vi "RT.vi"() -> ()   [LabVIEW 2014]
uses:
  <vilib>/NI/LVFPGA Adv Session Resources/OpenByNameSubVI.vi
  <vilib>/FPGAPlugInAG/Dynamic/niLvFpga_Run_Dynamic.vi
  <vilib>/rvi/interface/common/dynamic/niFpgaEscapeDelimiterAndNull.vi
  <vilib>/Utility/error.llb/Error Cluster From Error Code.vi
  <vilib>/rvi/errors/niLvFpgaAdjustHostInterfaceError.vi
  <vilib>/FPGAPlugInAG/Dynamic/niLvFpga_Close_Dynamic.vi
  <vilib>/rvi/interface/nirviMethod/nirviMethod.xnode
  <vilib>/NI/LVFPGA Adv Session Resources/OpenByName.xnode
  <vilib>/rvi/interface/nirviReadWriteControl/nirviReadWriteControl.xnode
  <vilib>/rvi/interface/nirviCloseFPGA/nirviCloseFPGA.xnode
  <vilib>/FPGAPlugInAG/Dynamic/niLvFpga_WriteFifo_Dynamic.vi
  <vilib>/rvi/errors/niLvFpgaMergeErrorWithErrorCode.vi
  <vilib>/NI/LVFPGA Adv Session Resources/LVFPGAAdvSessionResources.lvlib
  NiFpgaLv.dll
  <vilib>/rvi/interface/Simulation/niFpgaSimulationCallBeginRW.vi
panel:
  out "Value":u32 format="%x"
  in  "Bitfile path":path=path "c:/ni-rt/LabVIEW Data/DETSPIExample_FPGATarget_SPIperipheral_T23U1l-two8.lvbitx"
  out "Empty Elements Remaining":u32=16383
  out "error out":errorcluster={"status"=FALSE, "code"=61003, "source"="niLvFpga_Run_Dynamic.vi"}
  in  "SPI command":u32=589824 format="%x"
  in  "Boolean":bool
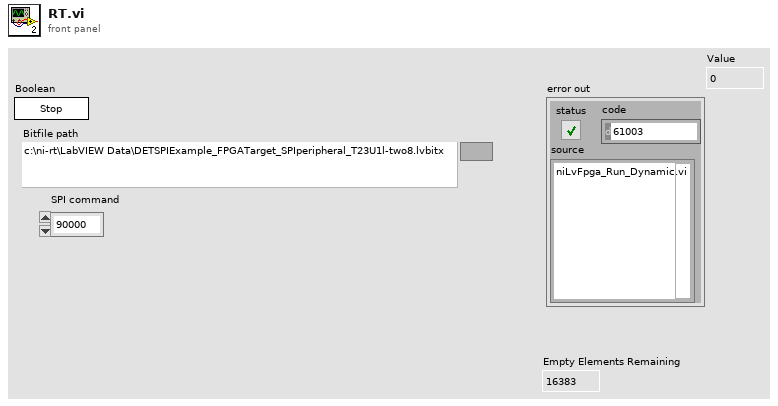
[diagram p1: front panel]
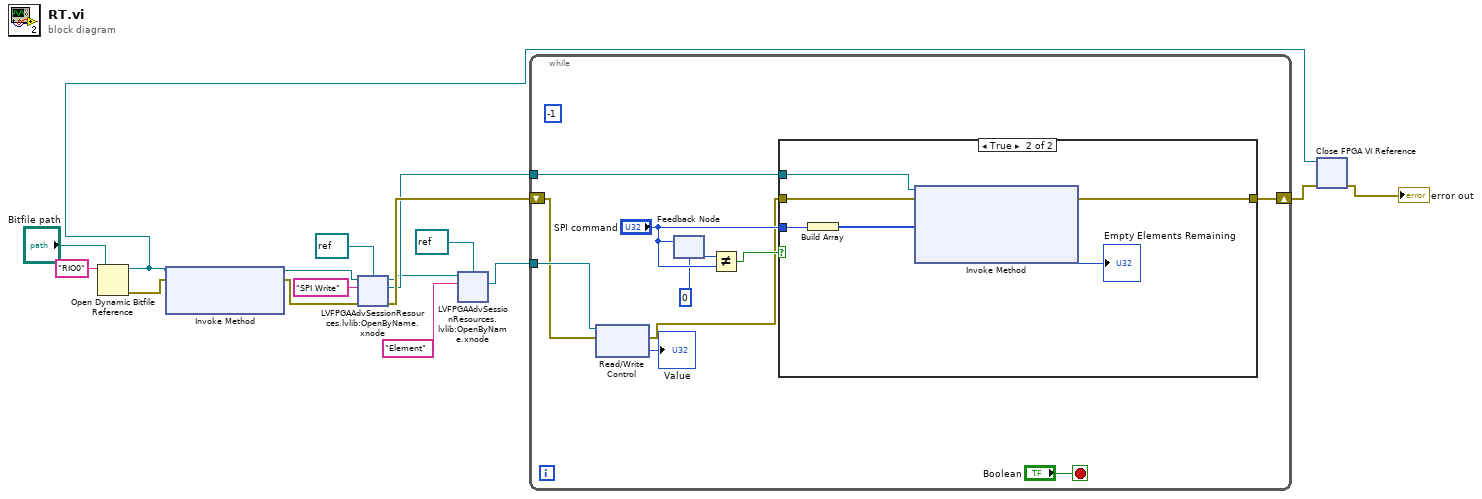
[diagram p0: block diagram]
diagram:
  n1 = Open Dynamic Bitfile Reference(0:"RIO0" ("Device address"), 1:"Bitfile path") -> (5:w11:refnum<k20>, 8:w14:errorcluster)  [unwired: 3 in]
  n2 = xnode "Invoke Method"("FPGA VI Reference In"=w11, "error in"=w14) -> ("FPGA VI Reference Out"=w5:refnum<k20>, "error out"=w8:errorcluster)  [unwired: 1 in]
  n3 = xnode "LVFPGAAdvSessionResources.lvlib:OpenByName.xnode"("FPGA VI Reference in"=w5, "Resource name in"="SPI Write", "Single resource reference type in"=refnum<k20> refnum, "Error in"=w8) -> ("Single resource reference out"=w6:refnum<k20>, "Error out"=w7:errorcluster, "FPGA VI Reference out"=w2:refnum<k20>)
  n4 = xnode "LVFPGAAdvSessionResources.lvlib:OpenByName.xnode"("FPGA VI Reference in"=w2, "Resource name in"="Element", "Single resource reference type in"=refnum<k20> refnum) -> ("Single resource reference out"=w1:refnum<k20>)  [unwired: 1 in, 2 out]
  n5 = while {
    tunnel: w6 -> [w21]
    shift-right: [w26] -> w13
    shift-left: w7 -> [w18]
    tunnel: w1 -> [w20]
    stop <- "Boolean" stop-if-true
    (unwired) -1
    n6 = xnode "Read/Write Control"("FPGA VI Reference In"=w20, "error in"=w18) -> ("error out"=w17:errorcluster, "Value"=→"Value":u32)  [unwired: 1 out]
    n7 = feedback-in #1("SPI command") -> ()
    n8 = feedback #1(u32 0 ("SPI command")) -> (w24:u32)
    n9 = Not Equal?(x=w24, y="SPI command") -> (x != y?=w22:bool)
    n10 = case shown="True" w22 {
      tunnel: w17 -> [w28 w32]
      tunnel: [w28 w31] -> w26
      tunnel: "SPI command" -> [_ w34]
      tunnel: w21 -> [_ w29]
      frame False {
      }
      frame True {
        n11 = Build Array(w34) -> (w33:u32[])
        n12 = xnode "Invoke Method"("FPGA VI Reference In"=w29, "error in"=w32, "Data"=w33) -> ("error out"=w31:errorcluster, "Empty Elements Remaining"=→"Empty Elements Remaining":u32)  [unwired: 1 in, 1 out]
      }
    }
  }
  n13 = xnode "Close FPGA VI Reference"("FPGA VI Reference In"=w11, "error in"=w13) -> ("error out"=→"error out":errorcluster)
